vi "initFileContentsTree.vi"(4 "error in (no error)":errorcluster, 5 "file path":path, 6 "Tree Refnum":refnum<vi>, 7 "tdms file":refnum<k34>) -> (0 "error out":errorcluster, 3 "tdms file out":refnum<k34>)   [LabVIEW 2015]
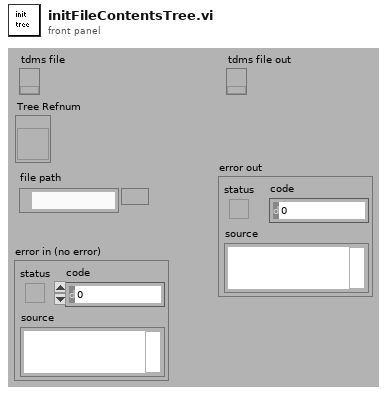
[diagram p1: front panel]
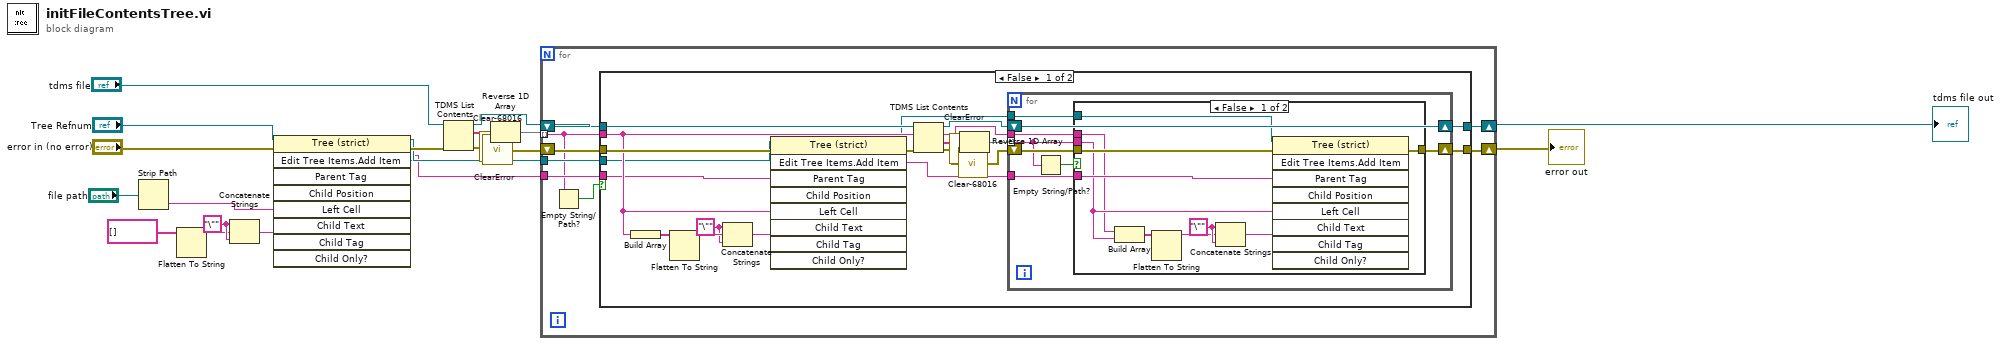
[diagram p0: block diagram]
diagram:
  w9 = "\"" ("string")
  n1 = Strip Path(path="file path") -> (name=w10:string)  [unwired: 1 out]
  n2 = Flatten To String(anything=string[] [] ("appended array")) -> (data string=w8:string)  [unwired: 3 in, 2 out]
  n3 = Concatenate Strings(w9, w8, w9) -> (w6:string)
  n4 = invoke on="Invoke Node" class="Tree (strict)" method="Edit Tree Items.Add Item"(reference="Tree Refnum", error in="error in (no error)", "Left Cell"=w10, "Child Tag"=w6) -> (reference out=w12:refnum<vi>, error out=w15:errorcluster, "Edit Tree Items:Add Item"=w5:string)  [unwired: 5 in, 6 out]
  n5 = TDMS List Contents(4:w15, 7:"tdms file") -> (0:w1:errorcluster, 2:w4:string[], 3:w16:refnum<k34>)  [unwired: 1 in, 1 out]
  n6 = call <vilib>:"ClearError.vi"("error in (no error)"=w1) -> ("error out"=w3:errorcluster)
  n7 = call <vilib>:"Clear-68016.vi"("error in (no error)"=w3) -> ("error out"=w2:errorcluster)
  n8 = Reverse 1D Array(array=w4) -> (reversed array=w18:string[])
  n9 = for {
    tunnel: w18 -> [w22] mode=indexing
    shift-right: [w25] -> w19
    shift-left: w16 -> [w27]
    shift-right: [w26] -> w20
    shift-left: w2 -> [w28]
    tunnel: w12 -> [w24]
    tunnel: w5 -> [w23]
    n10 = Empty String/Path?(string/path=w22) -> (empty?=w21:bool)
    n11 = case shown="False" w21 {
      tunnel: w28 -> [w49 w69]
      tunnel: w27 -> [w47 w70]
      tunnel: [w46 w69] -> w26
      tunnel: [w44 w70] -> w25
      tunnel: w22 -> [w42 _]
      tunnel: w24 -> [w35 _]
      tunnel: w23 -> [w33 _]
      frame False {
        w36 = "\"" ("string")
        n12 = Build Array(w42) -> (w41:string[])
        n13 = Flatten To String(anything=w41) -> (data string=w38:string)  [unwired: 3 in, 2 out]
        n14 = Concatenate Strings(w36, w38, w36) -> (w37:string)
        n15 = invoke on="Invoke Node" class="Tree (strict)" method="Edit Tree Items.Add Item"(reference=w35, error in=w49, "Parent Tag"=w33, "Left Cell"=w42, "Child Tag"=w37) -> (reference out=w34:refnum<vi>, error out=w48:errorcluster, "Edit Tree Items:Add Item"=w43:string)  [unwired: 4 in, 6 out]
        n16 = TDMS List Contents(4:w48, 6:w42, 7:w47) -> (0:w29:errorcluster, 1:w32:string[], 2:w40:string, 3:w45:refnum<k34>)
        n17 = call <vilib>:"ClearError.vi"("error in (no error)"=w29) -> ("error out"=w31:errorcluster)
        n18 = call <vilib>:"Clear-68016.vi"("error in (no error)"=w31) -> ("error out"=w30:errorcluster)
        n19 = Reverse 1D Array(array=w32) -> (reversed array=w39:string[])
        n20 = for {
          tunnel: w39 -> [w51] mode=indexing
          shift-right: [w55] -> w44
          shift-left: w45 -> [w55]
          shift-right: [w56] -> w46
          shift-left: w30 -> [w57]
          tunnel: w43 -> [w54]
          tunnel: w40 -> [w53]
          tunnel: w34 -> [w50]
          n21 = Empty String/Path?(string/path=w51) -> (empty?=w52:bool)
          n22 = case shown="False" w52 {
            tunnel: w57 -> [w67 w68]
            tunnel: [w66 w68] -> w56
            tunnel: w54 -> [w65 _]
            tunnel: w51 -> [w63 _]
            tunnel: w53 -> [w62 _]
            tunnel: w50 -> [w58 _]
            frame False {
              w61 = "\"" ("string")
              n23 = Build Array(w62, w63) -> (w64:string[])
              n24 = Flatten To String(anything=w64) -> (data string=w59:string)  [unwired: 3 in, 2 out]
              n25 = Concatenate Strings(w61, w59, w61) -> (w60:string)
              n26 = invoke on="Invoke Node" class="Tree (strict)" method="Edit Tree Items.Add Item"(reference=w58, error in=w67, "Parent Tag"=w65, "Left Cell"=w63, "Child Tag"=w60) -> (error out=w66:errorcluster)  [unwired: 4 in, 8 out]
            }
            frame True {
            }
          }
        }
      }
      frame True {
      }
    }
  }
  "error out" <- w20
  "tdms file out" <- w19
